vi "Save Setup.vi"(8 "error in (no error)":errorcluster, 10 "Memory Address(1-30)":i32=1, 11 "Visa Resource Name IN":refnum<visa-resource-name>) -> (0 "error out":errorcluster, 3 "Visa Resource Name OUT":refnum<visa-resource-name>)   [LabVIEW 2018, in "Keithley KE22xx Series.lvlib"]
doc: "To save the present settings of an instrument to specified memory location (1-30)."
uses:
  Keithley KE22xx Series.lvlib
panel:
  # "© 2012 Keithley Instruments, Inc. ALL RIGHTS RESERVED"
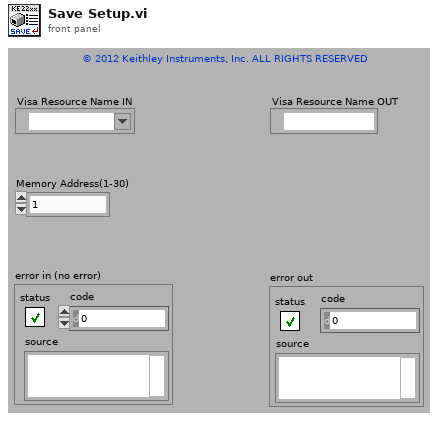
[diagram p1: front panel]
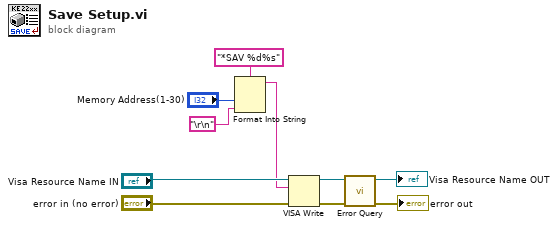
[diagram p0: block diagram]
diagram:
  n1 = Format Into String(format string="*SAV %d%s", "Memory Address(1-30)", "\r\n") -> (resulting string=w1:string)  [unwired: 2 in, 1 out]
  n2 = VISA Write(VISA resource name="Visa Resource Name IN", write buffer=w1, error in (no error)="error in (no error)") -> (VISA resource name out=w8:refnum<visa-resource-name>, error out=w7:errorcluster)  [unwired: 1 out]
  n3 = call "Error Query.vi"("error in (no error)"=w7, "VISA resource name"=w8) -> ("error out"=→"error out":errorcluster, "VISA resource name out"=→"Visa Resource Name OUT":refnum<visa-resource-name>)  [unwired: 6 in, 2 out]
